vi "GUILib.load and run.vi"(0 "path":string, 2 "userEvent":refnum<user-event>, 5 "error in (no error)":errorcluster, 7 "iniData":string) -> (14 "VIRef":refnum<vi>, 19 "error out":errorcluster)   [LabVIEW 2012, in "GUILib.lvlib"]
doc: "Opens a refnum to the specified VI and runs it."
uses:
  GUILib.lvlib
  GUILib.userEventsMainType.ctl
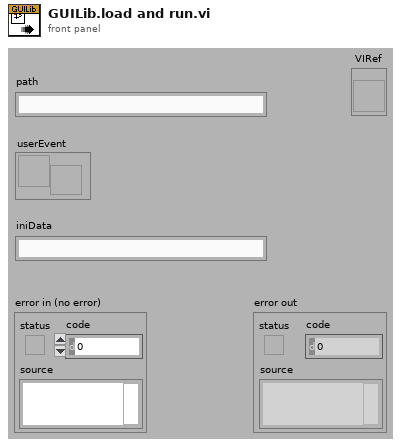
[diagram p1: front panel]
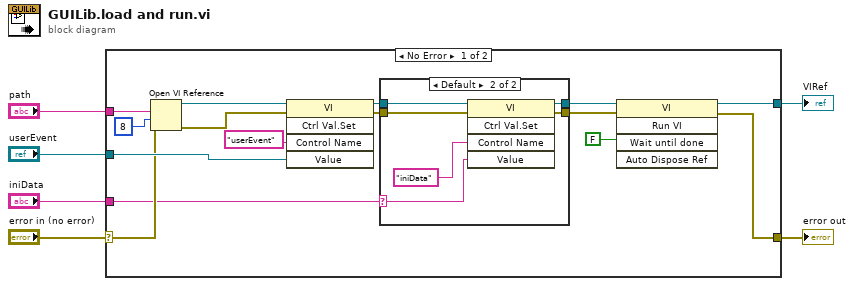
[diagram p0: block diagram]
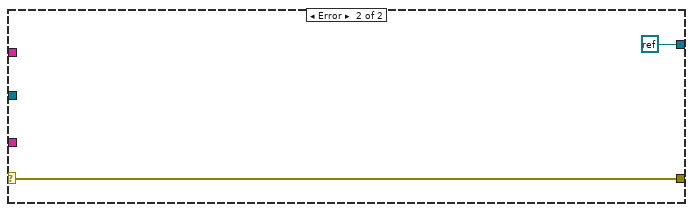
[diagram p3: hidden frame]
diagram:
  n1 = case shown="No Error" "error in (no error)" {
    selector: "error in (no error)" -> [w13 w30]
    tunnel: [w20 refnum<k0> refnum] -> w5
    tunnel: [w18 w30] -> w4
    tunnel: "path" -> [w15 _]
    tunnel: "userEvent" -> [w14 _]
    tunnel: "iniData" -> [w8 _]
    frame No Error {
      n2 = Open VI Reference(vi path=w15, options=8, error in (no error)=w13) -> (vi reference=w21:refnum<vi>, error out=w19:errorcluster)  [unwired: 3 in]
      n3 = invoke class="VI" method="Ctrl Val.Set"(reference=w21, error in=w19, "Control Name"="userEvent", "Value"=w14) -> (reference out=w12:refnum<vi>, error out=w11:errorcluster)  [unwired: 1 in, 3 out]
      n4 = case shown="Default" w8 {
        selector: w8 -> [_ w24]
        tunnel: w12 -> [w23 w29]
        tunnel: w11 -> [w22 w28]
        tunnel: [w23 w27] -> w10
        tunnel: [w22 w25] -> w9
        frame "", "N/A" {
        }
        frame Default {
          n5 = invoke class="VI" method="Ctrl Val.Set"(reference=w29, error in=w28, "Control Name"="iniData", "Value"=w24) -> (reference out=w27:refnum<vi>, error out=w25:errorcluster)  [unwired: 1 in, 3 out]
        }
      }
      n6 = invoke class="VI" method="Run VI"(reference=w10, error in=w9, "Wait until done"=FALSE) -> (reference out=w20:refnum<vi>, error out=w18:errorcluster)  [unwired: 2 in, 3 out]
    }
    frame Error {
    }
  }
  "VIRef" <- w5
  "error out" <- w4
